vi "has_state_changed.vi"() -> (0 "Just Exited Autonomous":bool, 1 "Just Entered Autonomous":bool, 2 "Just Disabled":bool, 3 "Just Enabled":bool)   [LabVIEW 2011]
uses:
  <vilib>/Rock Robotics/WPI/DriverStation/WPI_DriverStationCommDataCacheOp.ctl
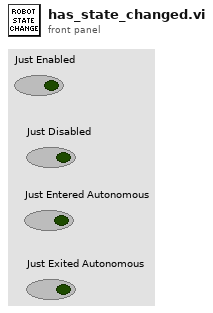
[diagram p1: front panel]
types:
  T1 = typedef "WPI_DriverStationCommDataCacheOp.ctl" = enum16{"Get", "Set", "Init"}
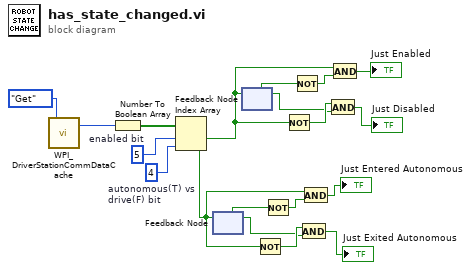
[diagram p0: block diagram]
diagram:
  w13 = 4  # autonomous(T) vs drive(F) bit
  w14 = 5  # enabled bit
  n1 = call <vilib>:"WPI_DriverStationCommDataCache.vi"("CommDataCacheOp"=WPI_DriverStationCommDataCacheOp."Get") -> ("ControlBit out"=w16:u8)  [unwired: 18 out]
  n2 = Number To Boolean Array(number=w16) -> (Boolean array=w15:bool[])
  n3 = Index Array(array=w15, index #1=w14, index #2=w13) -> (element #1=w10:bool, element #2=w1:bool)
  n4 = feedback #1() -> (w4:bool)  [unwired: 1 in]
  n5 = feedback-in #1(w1) -> ()
  n6 = feedback-in #2(w10) -> ()
  n7 = feedback #2() -> (w8:bool)  [unwired: 1 in]
  n8 = Not(x=w1) -> (.not. x?=w5:bool)
  n9 = Not(x=w4) -> (.not. x?=w6:bool)
  n10 = Not(x=w10) -> (.not. x?=w9:bool)
  n11 = Not(x=w8) -> (.not. x?=w12:bool)
  n12 = And(x=w5, y=w4) -> (x .and. y?=→"Just Exited Autonomous":bool)
  n13 = And(x=w1, y=w6) -> (x .and. y?=→"Just Entered Autonomous":bool)
  n14 = And(x=w9, y=w8) -> (x .and. y?=→"Just Disabled":bool)
  n15 = And(x=w10, y=w12) -> (x .and. y?=→"Just Enabled":bool)
